vi "Composite_Arithmatic.vi"() -> ()   [LabVIEW 2019]
panel:
  out "Result":dbl
  in  "int 4":dbl
  in  "int 3":dbl
  in  "int 2":dbl
  in  "int 1":dbl
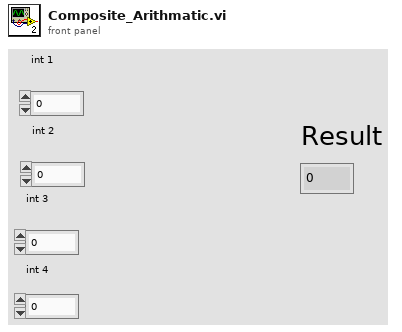
[diagram p1: front panel]
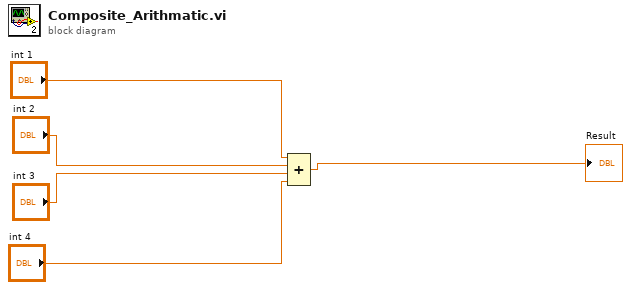
[diagram p0: block diagram]
diagram:
  n1 = Compound Arithmetic op=ADD("int 1", "int 2", "int 3", "int 4") -> (→"Result":dbl)
